vi "electrodes.vi"(4 "electrodes/ cell":i32=5, 6 "cell length (m)":dbl=0.02 format="%#_6p", 7 "phase / 2 pi":dbl, 9 "velocity":dbl[](array[numeric]), 10 "position":dbl[](array[numeric]), 11 "time":dbl[](array[numeric])) -> (2 "frequency":dbl[](array[numeric]), 3 "waveforms":dbl[][](array[numeric]))   [LabVIEW 2017, in "wf.lvlib" / "wf_tools.lvlib"]
uses:
  wf_tools.lvlib
panel:
  out "frequency t":cluster{"time":dbl[], dbl[]}(graph)
  out "frequency x":cluster{"position":dbl[], dbl[]}(graph)
  out "waveform x":cluster{"time":dbl[], dbl[]}[](graph)
  out "waveform t":cluster{"time":dbl[], dbl[]}[](graph)
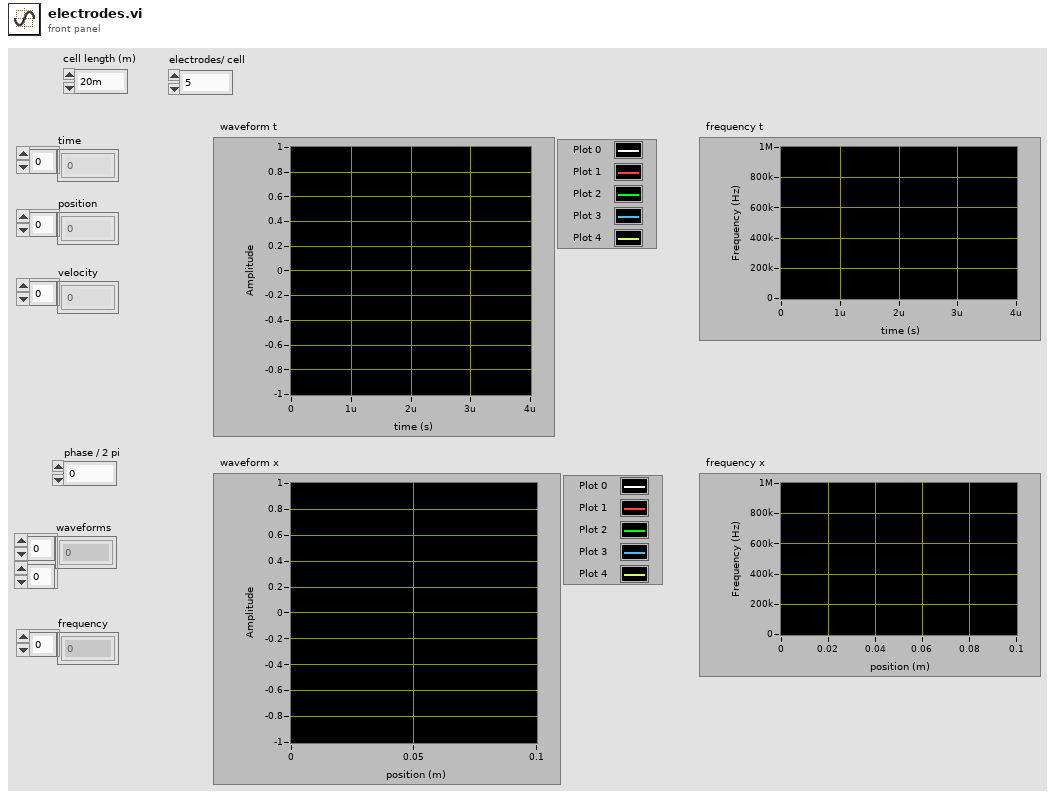
[diagram p1: front panel]
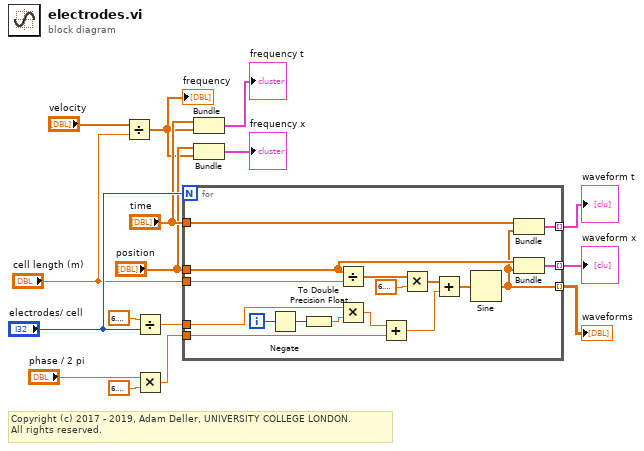
[diagram p0: block diagram]
diagram:
  # "Copyright (c) 2017 - 2019, Adam Deller, UNIVERSITY COLLEGE LONDON.\nAll rights reserved."
  n1 = Divide(x="velocity", y="cell length (m)") -> (x/y=w3:dbl[])
  "frequency" <- w3
  n2 = Divide(x=6.283185307179586, y="electrodes/ cell") -> (x/y=w14:dbl)
  n3 = Multiply(x="phase / 2 pi", y=6.283185307179586) -> (x*y=w6:dbl)
  n4 = for {
    N: "electrodes/ cell" -> [_]
    tunnel: w14 -> [w33]
    tunnel: "time" -> [w22]
    tunnel: "position" -> [w21]
    tunnel: "cell length (m)" -> [w23]
    tunnel: [w32] -> w9 mode=indexing
    tunnel: [w27] -> w10 mode=indexing
    tunnel: w6 -> [w25]
    tunnel: [w20] -> w5 mode=indexing
    i -> [w19]
    n5 = Negate(x=w19) -> (-x=w18:i32)
    n6 = To Double Precision Float(number=w18) -> (double precision float=w17:dbl)
    n7 = Divide(x=w21, y=w23) -> (x/y=w30:dbl[])
    n8 = Multiply(x=w33, y=w17) -> (x*y=w26:dbl)
    n9 = Add(x=w26, y=w25) -> (x+y=w24:dbl)
    n10 = Multiply(x=w30, y=6.283185307179586) -> (x*y=w28:dbl[])
    n11 = Add(x=w28, y=w24) -> (x+y=w31:dbl[])
    n12 = Sine(x=w31) -> (sin(x)=w20:dbl[])
    n13 = Bundle("time"=w22, w20) -> (w32:cluster{"time":dbl[], dbl[]})  [unwired: 1 in]
    n14 = Bundle("position"=w21, w20) -> (w27:cluster{"position":dbl[], dbl[]})  [unwired: 1 in]
  }
  "waveform t" <- w9
  "waveform x" <- w10
  "waveforms" <- w5
  n15 = Bundle("time"="time", w3) -> (→"frequency t":cluster{"time":dbl[], dbl[]})  [unwired: 1 in]
  n16 = Bundle("position"="position", w3) -> (→"frequency x":cluster{"position":dbl[], dbl[]})  [unwired: 1 in]
